vi "G#Object_Clear.vi"(5 "error in (no error)":errorcluster) -> (19 "error out":errorcluster)   [LabVIEW 2017, in "G#Object.lvclass"]
doc: "Clears all remaining queues and events used by the G# object lists. It also kills all class attributes queues and data value references as well as the external create process (if running)."
uses:
  G#Object.lvclass
  utils/G#Object_State.ctl
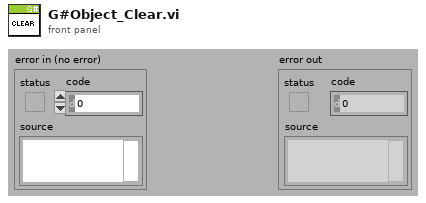
[diagram p1: front panel]
types:
  T1 = cluster{"queue name":string, "reference":refnum<class "G#Object.lvclass">}
  T2 = cluster{"queue name":string, "reference":refnum<class "G#Object.lvclass">}[]
  T3 = cluster{cluster{"queue name":string, "reference":refnum<class "G#Object.lvclass">}[]}[]
  T4 = typedef "G#Object.lvclass/G#Object_State.ctl" = enum16{"Clear", "Create", "Delete", "Get class attributes", "Class hierarchy", "Get attribute value", "Set attribute value"}
  T5 = cluster{cluster{"queue name":string, "reference":refnum<class "G#Object.lvclass">}[]}
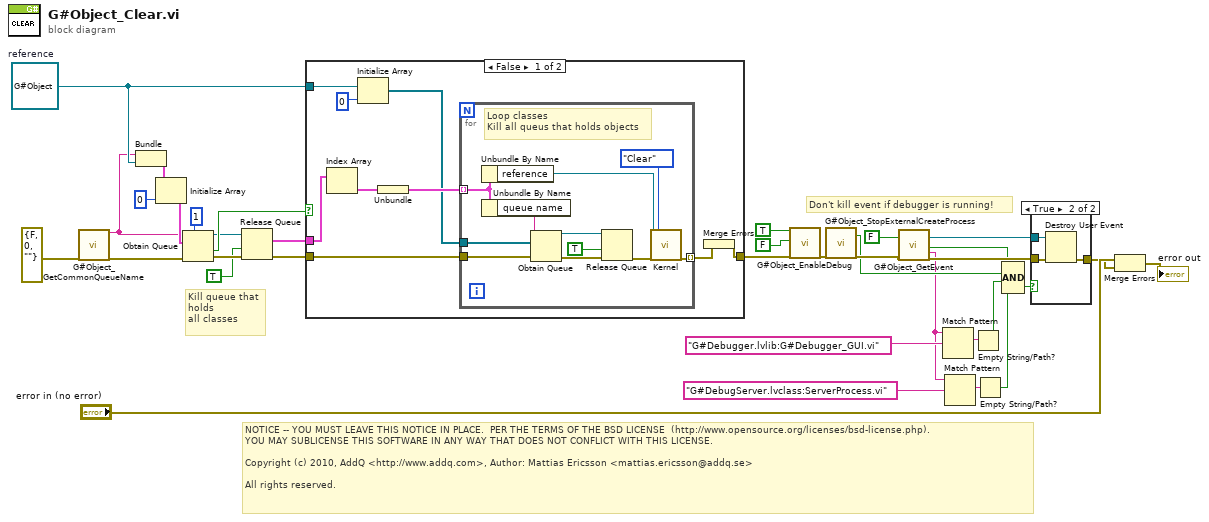
[diagram p0: block diagram]
diagram:
  w11 = refnum<class "G#Object.lvclass"> refnum  # reference
  # "NOTICE -- YOU MUST LEAVE THIS NOTICE IN PLACE.  PER THE TERMS OF THE BSD LICENSE  (http://www.opensource.org/licenses/bsd-license.php).\nYOU MAY SUBLICENSE THIS SOFTWARE IN ANY WAY THAT DOES NOT CONFLICT WITH THIS LICENSE.\n\nCopyright (c) 2010, AddQ <http://www.addq.com>, Author: Mattias Ericsson <mattias.ericsson@addq.se>\n\nAll rights reserved."
  # "Don't kill event if debugger is running!"
  # "Kill queue that\nholds\nall classes"
  n1 = call "G#Object_GetCommonQueueName.vi"("error in (no error)"=errorcluster {"status"=FALSE, "code"=0, "source"=""}) -> ("queue name"=w8:string, "error out"=w9:errorcluster)  [unwired: 17 in]
  n2 = Bundle("queue name"=w8, "reference"=w11) -> (w26:T1)  [unwired: 1 in]
  n3 = Initialize Array(w26, 0 ("dimension size")) -> (w25:T2)
  n4 = Obtain Queue(max queue size (-1, unlimited)=1, name (unnamed)=w8, element data type=w25, error in (no error)=w9) -> (queue out=w32:refnum<queue>, created new?=w35:bool, error out=w34:errorcluster)  [unwired: 1 in]
  n5 = Release Queue(queue=w32, force destroy? (F)=TRUE, error in (no error)=w34) -> (remaining elements=w30:T3, error out=w33:errorcluster)  [unwired: 1 out]
  n6 = case shown="False" w35 {
    tunnel: w33 -> [w43 w56]
    tunnel: [w40 w56] -> w13
    tunnel: w11 -> [w38 _]
    tunnel: w30 -> [w42 _]
    frame False {
      n7 = Index Array(array=w42) -> (element=w41:T5)  [unwired: 1 in]
      n8 = Initialize Array(w38, 0 ("dimension size")) -> (w37:refnum<class "G#Object.lvclass">[])
      n9 = Unbundle(w41) -> (w39:T2)
      n10 = for {
        tunnel: [w48] -> w44 mode=indexing
        tunnel: w43 -> [w52]
        tunnel: w37 -> [w51]
        tunnel: w39 -> [w46] mode=indexing
        # "Loop classes\nKill all queus that holds objects"
        n11 = Unbundle By Name(w46) -> ("reference"=w45:refnum<class "G#Object.lvclass">)
        n12 = Unbundle By Name(w46) -> ("queue name"=w50:string)
        n13 = Obtain Queue(name (unnamed)=w50, element data type=w51, error in (no error)=w52) -> (queue out=w55:refnum<queue>, error out=w54:errorcluster)  [unwired: 2 in, 1 out]
        n14 = Release Queue(queue=w55, force destroy? (F)=TRUE, error in (no error)=w54) -> (error out=w49:errorcluster)  [unwired: 2 out]
        n15 = call-dynamic "Kernel.vi"("reference in"=w45, "error in (no error)"=w49, "state"=G#Object_State."Clear" ("State")) -> ("error out"=w48:errorcluster)  [unwired: 8 in, 8 out]
      }
      n16 = Merge Errors(w44) -> (w40:errorcluster)
    }
    frame True {
    }
  }
  n17 = call "G#Object_EnableDebug.vi"("set (F)"=TRUE, "debug enable (F)"=FALSE, "error in (no error)"=w13) -> ("error out"=w14:errorcluster)  [unwired: 14 in, 2 out]
  n18 = call "G#Object_StopExternalCreateProcess.vi"("error in (no error)"=w14) -> ("stopped?"=w12:bool, "error out"=w17:errorcluster)  [unwired: 17 in]
  n19 = call "G#Object_GetEvent.vi"("create if needed (T)"=FALSE ("CreateIfNeeded"), "error in (no error)"=w17) -> ("G# event"=w23:refnum<user-event>, "valid"=w20:bool, "event owner"=w6:string, "error out"=w22:errorcluster)  [unwired: 13 in, 1 out]
  n20 = Match Pattern(string=w6, regular expression="G#Debugger.lvlib:G#Debugger_GUI.vi") -> (match substring=w4:string)  [unwired: 1 in, 3 out]
  n21 = Match Pattern(string=w6, regular expression="G#DebugServer.lvclass:ServerProcess.vi") -> (match substring=w2:string)  [unwired: 1 in, 3 out]
  n22 = Empty String/Path?(string/path=w4) -> (empty?=w3:bool)
  n23 = Empty String/Path?(string/path=w2) -> (empty?=w1:bool)
  n24 = Compound Arithmetic op=AND(w20, w12, w3, w1) -> (w19:bool)
  n25 = case shown="True" w19 {
    tunnel: w22 -> [w57 w60]
    tunnel: [w57 w58] -> w18
    tunnel: w23 -> [_ w59]
    frame False {
    }
    frame True {
      n26 = Destroy User Event(user event=w59, error in=w60) -> (error out=w58:errorcluster)
    }
  }
  n27 = Merge Errors("error in (no error)", w18) -> (→"error out":errorcluster)
